vi "macro_LinearFilter_ExecuteAVG.vi"   [LabVIEW 2019, in "Trajectory_Library.lvlib"]
uses:
  Trajectory_Library.lvlib
types:
  T1 = enum16{"Moving Average", "Low Pass 1st Order Butterworth", "Low Pass 2nd Order Butterworth", "High Pass 1st Order Butterworth", "High Pass 2nd Order Butterworth"}
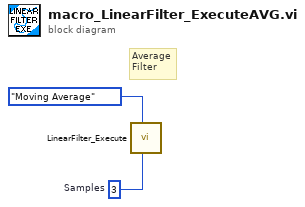
[diagram p0: block diagram]
diagram:
  w1 = 3  # Samples
  # "Average\nFilter"
  n1 = call "LinearFilter_Execute.vi"("Samples"=w1, "Filter Type"=T1."Moving Average") -> ()  [unwired: 8 in, 2 out]
